vi "Convert MC Event Increment.vi"(8 "error in (no error)":errorcluster, 10 "Event ID":T4(ring), 11 "ERD Data In":T3[](array[typedef]) {"ERD Number" format="%.0x"}) -> (0 "error out":errorcluster, 3 "Send ERD Data":T1[](array[typedef]) {"ERD Number" format="%.0x"})   [LabVIEW 2016, in "Centauro.lvlib"]
uses:
  Projects/Centauro.lvlib
  Common/LabVIEW GEA2 Toolkit/LabVIEW_GEA2_Toolkit.lvlibp/type defs/ERD Read Data Out.ctl
  Common/LabVIEW GEA2 Toolkit/LabVIEW_GEA2_Toolkit.lvlibp/type defs/ERD Write Data In.ctl
  Common/LabVIEW GEA2 Toolkit/LabVIEW_GEA2_Toolkit.lvlibp/type defs/Data Type.ctl
  Common/LabVIEW GEA2 Toolkit/LabVIEW_GEA2_Toolkit.lvlibp
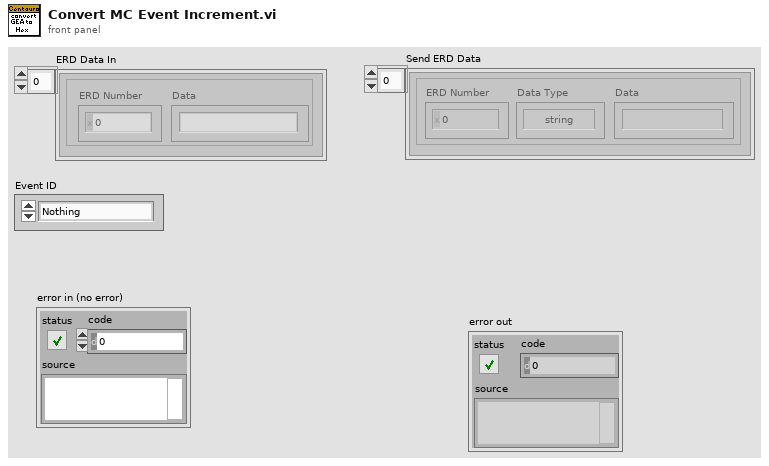
[diagram p1: front panel]
types:
  T1 = typedef "LabVIEW_GEA2_Toolkit.lvlibp/ERD Write Data In.ctl" = cluster{"ERD Number":u16, "Data Type":T2, "Data":string}
  T2 = typedef "LabVIEW_GEA2_Toolkit.lvlibp/Data Type.ctl" = enum16{"string", "boolean", "uint8_t", "uint16_t", "uint32_t", "uint64_t", "int8_t", "int16_t", "int32_t", "int64_t"}
  T3 = typedef "LabVIEW_GEA2_Toolkit.lvlibp/ERD Read Data Out.ctl" = cluster{"ERD Number":u16, "Data":string}
  T4 = enum16{"Nothing", "StartButtonPress", "StartButtonRelease", "DeepRinseKeyPress", "DeepRinseKeyRelease", "CycleKnobPosition0", "CycleKnobPosition1", "CycleKnobPosition2", "CycleKnobPosition3", "CycleKnobPosition4", "CycleKnobPosition5", "CycleKnobPosition6", "CycleKnobPosition7", "CycleKnobPosition8", "CycleKnobPosition9", "CycleKnobPosition10", "CycleKnobPosition11", "OptionKnob1Position0", "OptionKnob1Position1", "OptionKnob1Position2", "OptionKnob1Position3", "OptionKnob1Position4", "OptionKnob1Position5", "OptionKnob2Position0", "OptionKnob2Position1", "OptionKnob2Position2", "OptionKnob2Position3", "OptionKnob2Position4"}
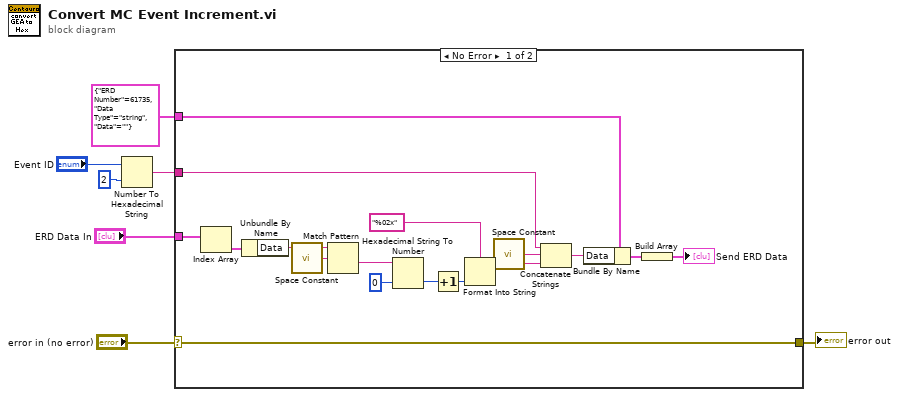
[diagram p0: block diagram]
diagram:
  n1 = Number To Hexadecimal String(1:i16 2 ("width (-)"), 2:"Event ID") -> (0:w2:string)
  n2 = case shown="No Error" "error in (no error)" {
    selector: "error in (no error)" -> [w11 w25]
    tunnel: [w11 w25] -> w6
    tunnel: "ERD Data In" -> [w10 _]
    tunnel: w2 -> [w9 _]
    tunnel: T1 {"ERD Number"=61735, "Data Type"=enum."string", "Data"=""} ("ERD Write Data In") -> [w8 _]
    frame No Error {
      n3 = Index Array(array=w10) -> (element=w15:T3)  [unwired: 1 in]
      n4 = Unbundle By Name(w15) -> ("Data"=w16:string)
      n5 = call <vilib>:"Space Constant.vi"() -> ("String"=w23:string)
      n6 = Match Pattern(string=w16, regular expression=w23) -> (after substring=w17:string)  [unwired: 1 in, 3 out]
      n7 = Hexadecimal String To Number(string=w17, default (0uL)=u8 0 ("default (0 U32)")) -> (number=w18:u8)  [unwired: 1 in, 1 out]
      n8 = Increment(x=w18) -> (x+1=w20:u8)
      n9 = Format Into String(format string="%02x", w20) -> (resulting string=w19:string)  [unwired: 2 in, 1 out]
      n10 = call <vilib>:"Space Constant.vi"() -> ("String"=w24:string)
      n11 = Concatenate Strings(w9, w24, w19) -> (w14:string)
      n12 = Bundle By Name(cluster=w8, "Data"=w14) -> (w13:T1)
      n13 = Build Array(w13) -> (→"Send ERD Data":T1[])
    }
    frame Error {
    }
  }
  "error out" <- w6
